vi "Voltage to Angle.vi"(7 "Numeric":dbl) -> (8 "Numeric 2":dbl)   [LabVIEW 2011]
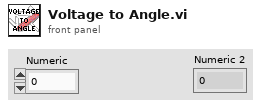
[diagram p1: front panel]
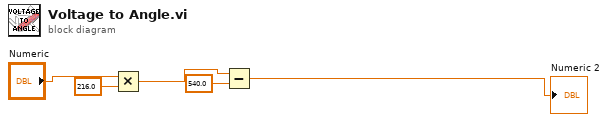
[diagram p0: block diagram]
diagram:
  n1 = Multiply(x="Numeric", y=216.0) -> (x*y=w2:dbl)
  n2 = Subtract(x=w2, y=540.0) -> (x-y=→"Numeric 2":dbl)
